vi "_FPGA Write Data.vi"(4 "Write Mode (Do Write)":T1=enum."Do Write", 5 "error in":errorcluster, 6 "Data":u32, 7 "Address":u16) -> (0 "error out":errorcluster)   [LabVIEW 2015]
uses:
  Type/_RW Status.ctl
  Type/_FPGA Indicator.ctl
  _RT Global.vi
  <vilib>/Utility/error.llb/Error Cluster From Error Code.vi
  <vilib>/rvi/errors/niLvFpgaAdjustHostInterfaceError.vi
  <vilib>/rvi/interface/nirviReadWriteControl/nirviReadWriteControl.xnode
  Type/FPGA Typedef.ctl
  FPGA Bitfiles/FPGA9607.lvbitx
  NiFpgaLv.dll
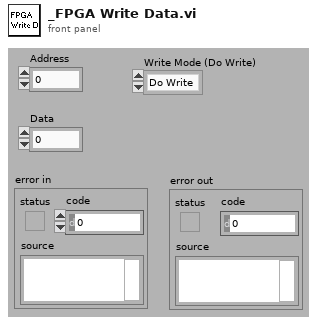
[diagram p1: front panel]
types:
  T1 = typedef "_RW Status.ctl" = enum8{"Done", "Do Read", "Do Write", "Set Latch1", "Set Latch2", "Set Latch3", "Set Latch4", "RP ON", "EL ON", "Serial Send", "Set LC Out", "Get LC In", "Read VAC", "Table Test", "Get Interlock", "Do Read2", "Do Write2"}
  T2 = typedef "Semaphore RefNum" = refnum<k1>
  T3 = typedef "_FPGA Indicator.ctl" = enum16{"Done", "Ready", "Count Available", "SendSerial", "LED State"}
  T4 = typedef "FPGA Typedef.ctl" = refnum<k20>
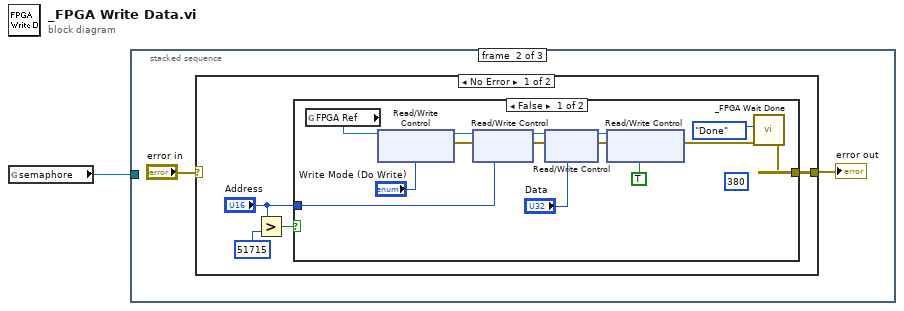
[diagram p0: block diagram]
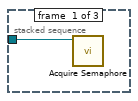
[diagram p2: hidden frame]
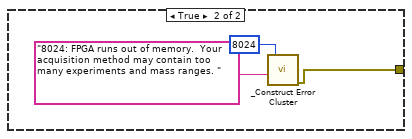
[diagram p3: hidden frame]
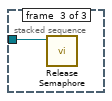
[diagram p5: hidden frame]
diagram:
  n1 = global read "_RT Global.vi" "semaphore"() -> (w1:T2)
  n2 = stacked-sequence {
    tunnel: w1 -> [w2 _ w27]
    frame #0 {
      n3 = call <vilib>:"Acquire Semaphore.vi"("semaphore"=w2) -> ()  [unwired: 2 in, 5 out]
    }
    frame #1 {
      n4 = case shown="No Error" "error in" {
        selector: "error in" -> [_ w26]
        tunnel: [w8 w26] -> w3
        frame No Error {
          n5 = Greater?(x="Address", y=u16 51715) -> (0:w5:bool)
          n6 = case shown="False" w5 {
            tunnel: [w9 w25] -> w8
            tunnel: "Address" -> [w11 _]
            frame False {
              (unwired) u32 380 ("Timeout (2000ms)")
              n7 = global read "_RT Global.vi" "FPGA Ref"() -> (w10:T4)
              n8 = xnode "Read/Write Control"("FPGA VI Reference In"=w10, "R/W Status"="Write Mode (Do Write)") -> ("FPGA VI Reference Out"=w15:T4, "error out"=w16:errorcluster)  [unwired: 1 in]
              n9 = xnode "Read/Write Control"("FPGA VI Reference In"=w15, "error in"=w16, "Address"=w11) -> ("FPGA VI Reference Out"=w17:T4, "error out"=w18:errorcluster)
              n10 = xnode "Read/Write Control"("FPGA VI Reference In"=w17, "error in"=w18, "Data"="Data") -> ("FPGA VI Reference Out"=w19:T4, "error out"=w20:errorcluster)
              n11 = xnode "Read/Write Control"("FPGA VI Reference In"=w19, "error in"=w20, "Read/Write"=TRUE ("Data Written")) -> ("error out"=w12:errorcluster)  [unwired: 1 out]
              n12 = call "_FPGA Wait Done.vi"("error in"=w12, "Indicator"=_FPGA_Indicator."Done") -> ("error out"=w9:errorcluster)  [unwired: 3 in, 2 out]
            }
            frame True {
              n13 = call "_Construct Error Cluster.vi"("reason"="8024: FPGA runs out of memory.  Your acquisition method may contain too many experiments and mass ranges. ", "errorCode"=8024) -> ("error out"=w25:errorcluster)  [unwired: 2 in, 3 out]
            }
          }
        }
        frame Error {
        }
      }
      "error out" <- w3
    }
    frame #2 {
      n14 = call <vilib>:"Release Semaphore.vi"("semaphore"=w27) -> ()  [unwired: 1 in, 6 out]
    }
  }
